vi "RB2 base station main demo 2.vi"() -> ()   [LabVIEW 2012]
panel:
  out "dot location string":string
  out "Dot Array":T1(array[cluster])
  out "All Found?":bool
  in  "stop":bool
  out "Mars image":T2(plugin-control)
  in  "Image file name":string="all dots 1.bmp"
  out "error out":errorcluster
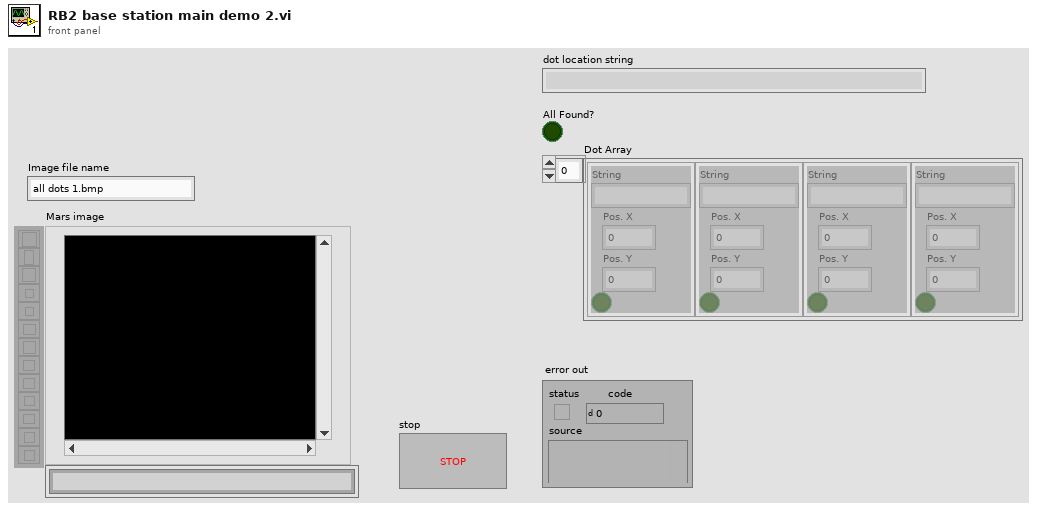
[diagram p1: front panel]
types:
  T1 = cluster{"String":string, "Pos. X":i32, "Pos. Y":i32, bool}[]
  T2 = typedef "IMAQ Image.ctl" = refnum<image>
  T3 = typedef "Image Type" = u32
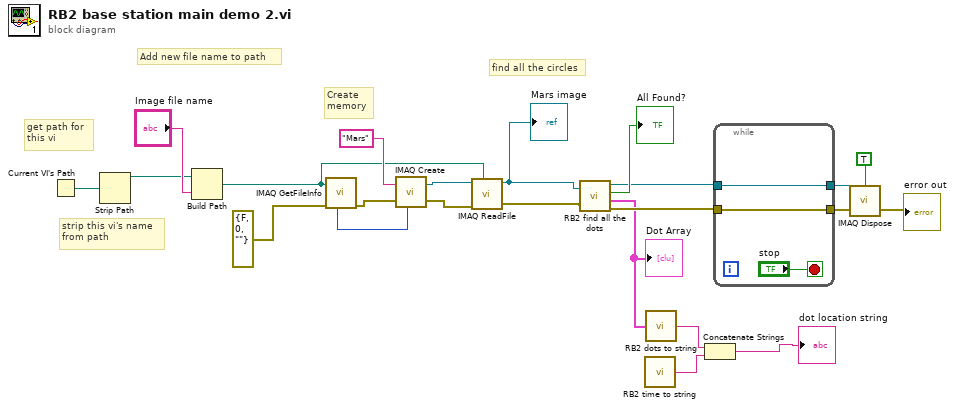
[diagram p0: block diagram]
diagram:
  # "find all the circles"
  # "Add new file name to path"
  # "strip this vi's name \nfrom path"
  # "get path for \nthis vi"
  # "Create \nmemory"
  n1 = Current VI's Path() -> (path=w18:path)
  n2 = Strip Path(path=w18) -> (stripped path=w17:path)  [unwired: 1 out]
  n3 = Build Path(base path=w17, name or relative path="Image file name") -> (appended path=w16:path)
  n4 = call "IMAQ GetFileInfo"("error in (no error)"=errorcluster {"status"=FALSE, "code"=0, "source"=""}, "File Path"=w16) -> ("error out"=w23:errorcluster, "Image Type"=w12:T3)  [unwired: 3 in, 5 out]
  n5 = call "IMAQ Create"("Image Name"="Mars", "Image Type"=w12, "error in (no error)"=w23) -> ("New Image"=w13:T2, "error out"=w20:errorcluster)  [unwired: 2 in]
  n6 = call "IMAQ ReadFile"("File Path"=w16, "error in (no error)"=w20, "Image"=w13) -> ("error out"=w8:errorcluster, "Image Out"=w9:T2)  [unwired: 4 in, 3 out]
  "Mars image" <- w9
  n7 = call "RB2 find all the dots.vi"("Image In"=w9, "error in"=w8) -> ("Image Out"=w6:T2, "All Found?"=→"All Found?":bool, "Dot Array"=w4:T1, "error out"=w5:errorcluster)
  "Dot Array" <- w4
  n8 = call "RB2 time to string.vi"() -> ("time string"=w2:string)  [unwired: 1 in]
  n9 = call "RB2 dots to string.vi"("Dot Array"=w4) -> ("dot location string"=w3:string)
  n10 = Concatenate Strings(w3, w2) -> (→"dot location string":string)
  n11 = while {
    tunnel: w6 -> [w25]
    tunnel: w5 -> [w24]
    tunnel: [w25] -> w11
    tunnel: [w24] -> w10
    stop <- "stop" stop-if-true
  }
  n12 = call "IMAQ Dispose"("All Images? (No)"=TRUE, "Image"=w11, "error in (no error)"=w10) -> ("error out"=→"error out":errorcluster)  [unwired: 3 in]
